vi "GasteilerStringLaden.vi"(11 "Array (Eingang)":string[][](array[string])) -> (2 "string array":string[][](array[string]), 3 "Cluster Array (Ausgang)":T1[](array[typedef]) {"Gasteiler Letzte Wartung" format="%<%x %.3X>T"})   [LabVIEW 2020, in "System Einstellungen V2.lvlib"]
uses:
  System Einstellungen V2.lvlib
  Gasteiler.ctl
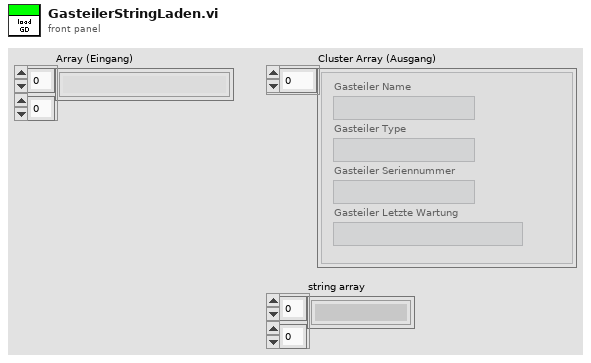
[diagram p1: front panel]
types:
  T1 = typedef "System Einstellungen V2.lvlib/Gasteiler.ctl" = cluster{"Gasteiler Name":string, "Gasteiler Type":string, "Gasteiler Seriennummer":string, "Gasteiler Letzte Wartung":timestamp}
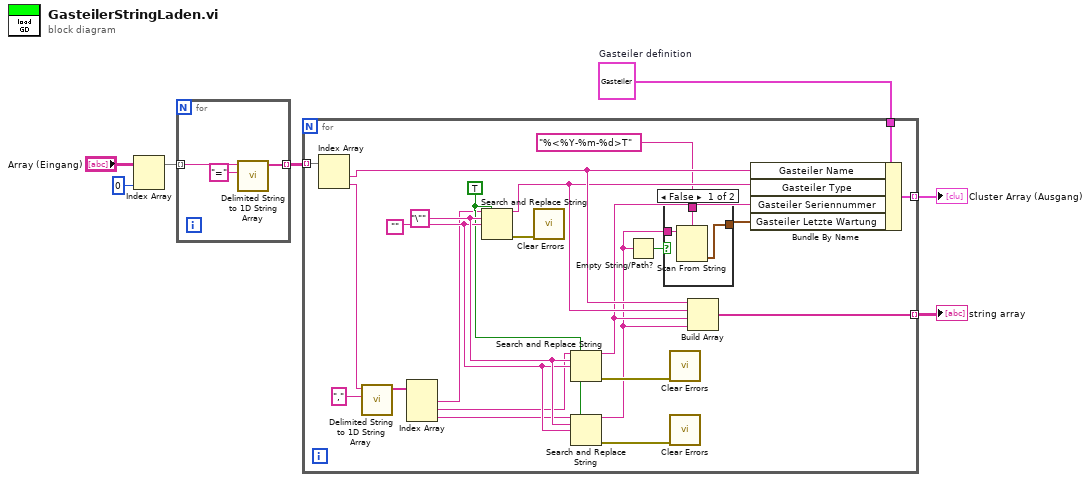
[diagram p0: block diagram]
diagram:
  w1 = T1 {"Gasteiler Name"="", "Gasteiler Type"="", "Gasteiler Seriennummer"="", "Gasteiler Letzte Wartung"=timestamp(0 s since 1904-01-01)}  # Gasteiler definition
  n1 = Index Array(array="Array (Eingang)", index (col)=0 ("Deaktivierter Index (Spalte)")) -> (element=w5:string[])  [unwired: 1 in]
  n2 = for {
    tunnel: w5 -> [w10] mode=indexing
    tunnel: [w8] -> w4 mode=indexing
    n3 = call <vilib>:"Delimited String to 1D String Array.vi"("delimiter"="=", "delimited string"=w10) -> ("string array"=w8:string[])  [unwired: 9 in]
  }
  n4 = for {
    tunnel: w4 -> [w32] mode=indexing
    tunnel: w1 -> [w33]
    tunnel: [w31] -> w7 mode=indexing
    tunnel: [w27] -> w3 mode=indexing
    w21 = ""
    w17 = TRUE ("Alle ersetzen? (F)")
    w22 = "\"" ("Such-String")
    n5 = Index Array(array=w32) -> (element #1=w29:string, element #2=w12:string)  [unwired: 2 in]
    n6 = call <vilib>:"Delimited String to 1D String Array.vi"("delimiter"="," ("Such-String/-Zeichen (-)"), "delimited string"=w12) -> ("string array"=w23:string[])  [unwired: 9 in]
    n7 = Index Array(array=w23) -> (element #1=w11:string, element #2=w13:string, element #3=w14:string)  [unwired: 3 in]
    n8 = Search and Replace String(replace all?=w17, input string=w11, search string=w22, replace string=w21) -> (result string=w28:string, error out=w30:errorcluster)  [unwired: 4 in, 2 out]
    n9 = call <vilib>:"Clear Errors.vi"("error in (no error)"=w30) -> ()  [unwired: 5 in, 2 out]
    n10 = Search and Replace String(replace all?=w17, input string=w13, search string=w22, replace string=w21) -> (result string=w25:string, error out=w26:errorcluster)  [unwired: 4 in, 2 out]
    n11 = Search and Replace String(replace all?=w17, input string=w14, search string=w22, replace string=w21) -> (result string=w15:string, error out=w20:errorcluster)  [unwired: 4 in, 2 out]
    n12 = Empty String/Path?(string/path=w15) -> (empty?=w16:bool)
    n13 = case shown="False" w16 {
      tunnel: w15 -> [w36 _]
      tunnel: "%<%Y-%m-%d>T" ("Format-String") -> [w35 _]
      tunnel: [w34 _] -> w18
      frame False {
        n14 = Scan From String(format string=w35, input string=w36) -> (output 1=w34:timestamp)  [unwired: 3 in, 3 out]
      }
      frame True {
      }
    }
    n15 = call <vilib>:"Clear Errors.vi"("error in (no error)"=w26) -> ()  [unwired: 5 in, 2 out]
    n16 = call <vilib>:"Clear Errors.vi"("error in (no error)"=w20) -> ()  [unwired: 5 in, 2 out]
    n17 = Build Array(w29, w28, w25, w15) -> (w27:string[])
    n18 = Bundle By Name(cluster=w33, "Gasteiler Name"=w29, "Gasteiler Type"=w28, "Gasteiler Seriennummer"=w25, "Gasteiler Letzte Wartung"=w18) -> (w31:T1)
  }
  "Cluster Array (Ausgang)" <- w7
  "string array" <- w3
